vi "Main.vi"() -> ()   [LabVIEW 2018]
uses:
  <vilib>/MakerHub/LINX/Public/Peripherals/PWM/PWM Set Duty Cycle N Chans.vi
  <vilib>/MakerHub/LINX/Public/Utilities/Open Serial.vi
  <vilib>/MakerHub/LINX/Public/Peripherals/PWM/PWM Set Duty Cycle 1 Chan.vi
  <vilib>/MakerHub/LINX/LMH-LINX.lvlib
panel:
  in  "Brightness":dbl(knob) scale=0.0..1.0
  in  "Baud Rate":u32=9600
  in  "?":bool
  out "error out":errorcluster
  in  "Serial Port":refnum<visa-resource-name>="N/A"
  # "Arduino Settings"
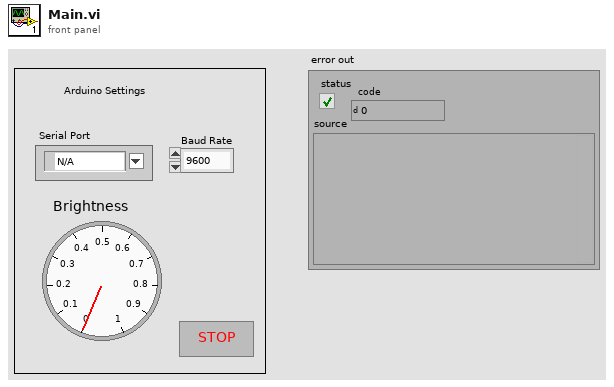
[diagram p1: front panel]
types:
  T1 = typedef "LMH-LINX.lvlib/LINX Ref.ctl" = cluster{"IO":T2, "Interface":T3, "LINX Device Config":T4}
  T2 = typedef "LMH-LINX.lvlib/Platform.ctl" = enum16{"Remote", "Local"}
  T3 = typedef "LMH-LINX.lvlib/Interface.ctl" = enum16{"Serial", "TCP"}
  T4 = typedef "LMH-LINX.lvlib/Device.lvlib/LINX Device Config.ctl" = cluster{"Interface":T3, "COM Port":refnum<visa-resource-name>, "TCP Configuration":T5, "Device Family":u8, "Device ID":u8, "Device Name":string, "TCP Ref":refnum<k5>, "Channels":T6}
  T5 = typedef "LMH-LINX.lvlib/Device.lvlib/TCP Config.ctl" = cluster{"IP Address":string, "Port":u16}
  T6 = typedef "LMH-LINX.lvlib/Channels.ctl" = cluster{"DI":u8[], "DO":u8[], "AI":u8[], "AO":u8[], "PWM":u8[], "QE":u8[], "UART":u8[], "I2C 2":u8[], "SPI":u8[], "CAN":u8[], "Servo":u8[], "AI Ref (V)":dbl, "AI Resolution (Bits)":u8, "AO Ref (V)":dbl, "AO Resolution (Bits)":u8}
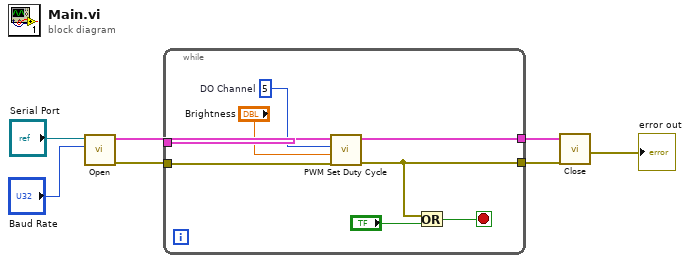
[diagram p0: block diagram]
diagram:
  n1 = call-poly <vilib>:"Open.vi"("Baud Rate Override"="Baud Rate", "Serial Port"="Serial Port") -> ("Error Out"=w3:errorcluster, "LINX Resource"=w4:T1)  [unwired: 7 in, 1 out]
  n2 = while {
    tunnel: w4 -> [w15]
    tunnel: w3 -> [w13]
    tunnel: [w14] -> w2
    tunnel: [w10] -> w1
    stop <- w9 stop-if-true
    w12 = u8 5  # DO Channel
    n3 = call-poly <vilib>:"PWM Set Duty Cycle.vi"("Error In"=w13, "Duty Cycle (0-1)"="Brightness", "PWM Channel"=w12, "LINX Resource"=w15) -> ("Error Out"=w10:errorcluster, "LINX Resource"=w14:T1)  [unwired: 6 in]
    n4 = Or(x=w10, y="?") -> (x .or. y?=w9:bool)
  }
  n5 = call <vilib>:"Close.vi"("Error In"=w1, "LINX Resource"=w2) -> ("Error Out"=→"error out":errorcluster)  [unwired: 9 in]
